vi "PRUEBA_DIG.vi"() -> ()   [LabVIEW 2025]
panel:
  in  "error in (no error)":errorcluster
  out "error out":errorcluster
  in  "stop":bool
  in  "Pin W":u8=4 min=4 max=40
  out "Valor":bool
  in  "Pin":u8=4 min=4 max=40
  in  "VISA resource name":refnum<visa-resource-name>
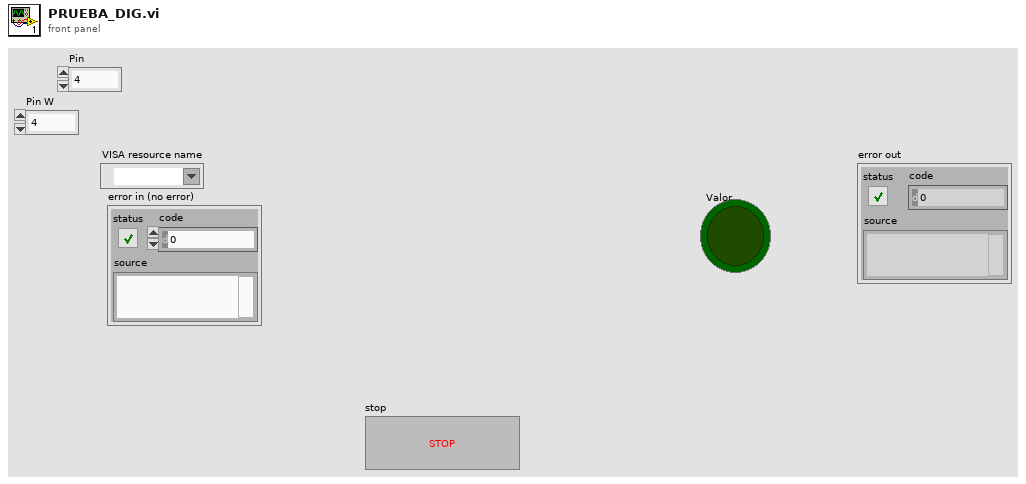
[diagram p1: front panel]
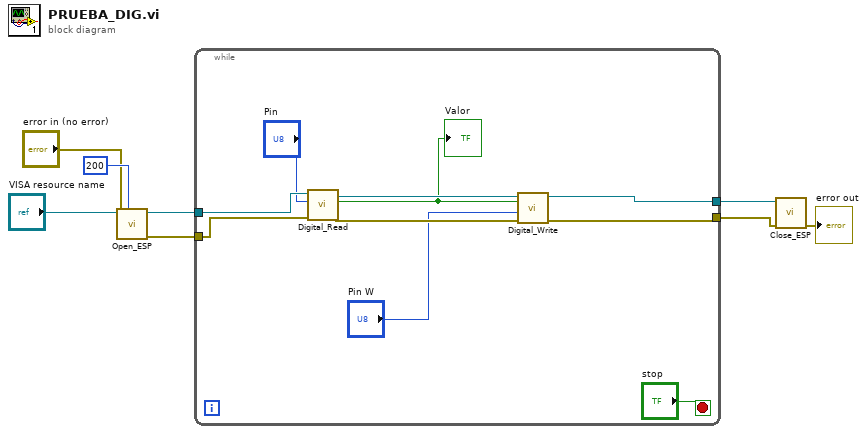
[diagram p0: block diagram]
diagram:
  n1 = call "Open_ESP.vi"("timeout (10sec)"=u32 200, "error in (no error)"="error in (no error)", "VISA resource name"="VISA resource name") -> ("error out"=w6:errorcluster, "VISA resource name out"=w7:refnum<visa-resource-name>)  [unwired: 7 in]
  n2 = while {
    tunnel: w7 -> [w18]
    tunnel: w6 -> [w11]
    tunnel: [w16] -> w4
    tunnel: [w15] -> w3
    stop <- "stop" stop-if-true
    n3 = call "Digital_Read.vi"("error in (no error)"=w11, "Pin"="Pin", "VISA resource name"=w18) -> ("error out"=w14:errorcluster, "Valor"=w9:bool, "VISA resource name out"=w13:refnum<visa-resource-name>)  [unwired: 6 in]
    "Valor" <- w9
    n4 = call "Digital_Write.vi"("error in (no error)"=w14, "Pin"="Pin W", "Estado"=w9, "VISA resource name"=w13) -> ("error out"=w15:errorcluster, "VISA resource name out"=w16:refnum<visa-resource-name>)  [unwired: 6 in]
  }
  n5 = call "Close_ESP.vi"("error in (no error)"=w3, "VISA resource name"=w4) -> ("error out"=→"error out":errorcluster)  [unwired: 9 in]
